vi "SetClockParameters.vi"(7 "ClockEnable":bool, 8 "error in (no error)":errorcluster, 9 "DivideBy":u32=8, 10 "ClockSource":T1=1 items=["Internal Oscillator"=1, "External Trigger"=2, "Trigger & Oscillator"=3, "MasterSlave Bus"=4], 11 "BME_DG_Base in":refnum<class "BME_DG_Base.lvclass">) -> (0 "error out":errorcluster, 3 "BME_DG_Base out":refnum<class "BME_DG_Base.lvclass">)   [LabVIEW 2009, in "BME_DG_Base.lvclass"]
uses:
  BME_DG_Base.lvclass
  LV-BME Interface/ClockSource.ctl
  BME_DG_Base.lvclass/BME_DG_Base.ctl
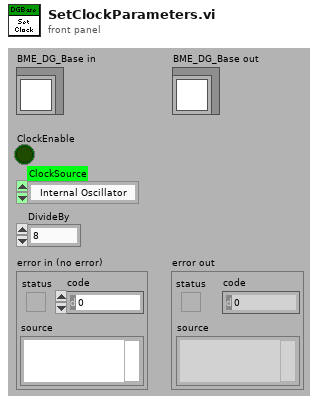
[diagram p1: front panel]
types:
  T1 = typedef "ClockSource.ctl" = i32
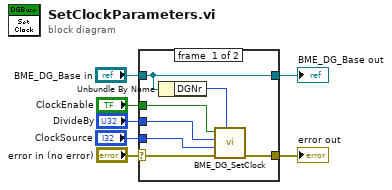
[diagram p0: block diagram]
diagram:
  n1 = case shown="No Error" "error in (no error)" {
    selector: "error in (no error)" -> [w12 w16]
    tunnel: [w11 w16] -> w6
    tunnel: [w14 w15] -> w4
    tunnel: "BME_DG_Base in" -> [w14 w15]
    tunnel: "ClockEnable" -> [w10 _]
    tunnel: "DivideBy" -> [w9 _]
    tunnel: "ClockSource" -> [w8 _]
    frame #0 {
      n2 = Unbundle By Name(w14) -> ("DGNr"=w13:i32)
      n3 = call "BME_DG_SetClock.vi"("DG_NumberM"=w13, "error in (no error)"=w12, "ClockSource"=w8, "DivideBy"=w9, "ClockEnable"=w10) -> ("error out"=w11:errorcluster)  [unwired: 5 in, 1 out]
    }
    frame #1 {
    }
  }
  "error out" <- w6
  "BME_DG_Base out" <- w4
